vi "Stop Reading.vi"(8 "error in (no error)":errorcluster, 11 "uCAN in":refnum<class "uCAN.lvclass">) -> (0 "error out":errorcluster, 3 "uCAN out":refnum<class "uCAN.lvclass">)   [LabVIEW 2021, in "uCanDriver.lvlib" / "uCAN.lvclass"]
uses:
  uCAN.lvclass
  typedefs/frame.ctl
  uCAN.lvclass/uCAN.ctl
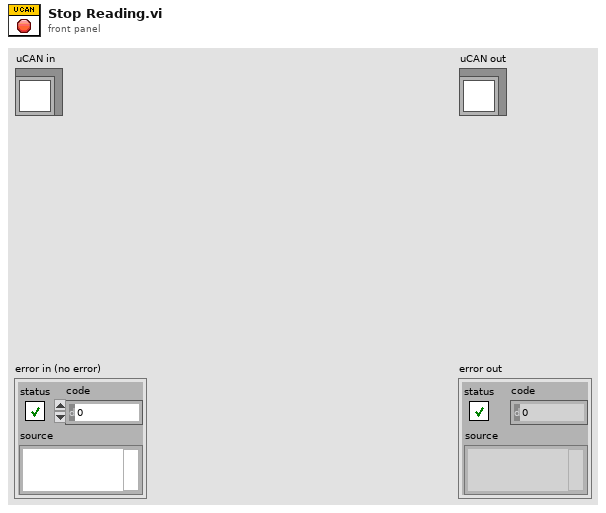
[diagram p1: front panel]
types:
  T1 = typedef "uCanDriver.lvlib/uCAN.lvclass/frame.ctl" = cluster{"Extended":bool, "ID":u32, "Data":u8[], "DLC":u8}
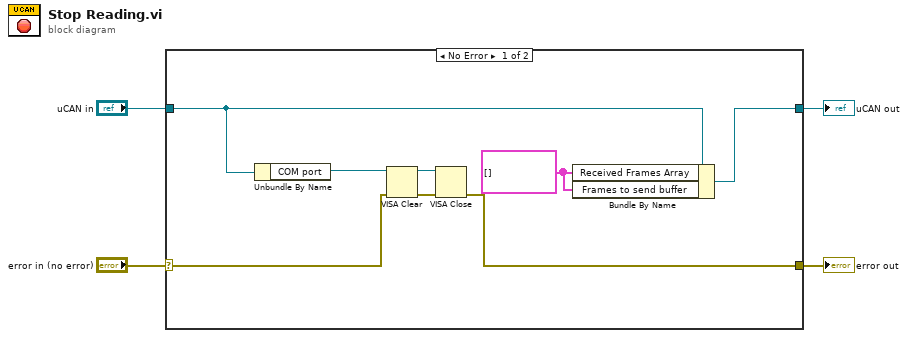
[diagram p0: block diagram]
diagram:
  n1 = case shown="No Error" "error in (no error)" {
    selector: "error in (no error)" -> [w8 w14]
    tunnel: [w7 w14] -> w3
    tunnel: [w6 w13] -> w1
    tunnel: "uCAN in" -> [w12 w13]
    frame No Error {
      w5 = T1[] [] ("Received Frames Array")
      n2 = Unbundle By Name(w12) -> ("COM port"=w11:refnum<visa-resource-name>)
      n3 = VISA Clear(VISA resource name=w11, error in (no error)=w8) -> (VISA resource name out=w10:refnum<visa-resource-name>, error out=w9:errorcluster)
      n4 = VISA Close(VISA resource name=w10, error in (no error)=w9) -> (error out=w7:errorcluster)
      n5 = Bundle By Name(cluster=w12, "Received Frames Array"=w5, "Frames to send buffer"=w5) -> (w6:refnum<class "uCAN.lvclass">)
    }
    frame Error {
    }
  }
  "error out" <- w3
  "uCAN out" <- w1
